vi "Init Master Slave Drive.vi"(0 "RobotDriveDevRef":T1={"DevStatus"={"status"=FALSE, "code"=0, "source"=""}, "Motors[]"=[], "Square Inputs"=FALSE, "Max Output"=1.0, "Isochronous"=FALSE}, 1 "Encoder Codes Per Rev":u16=64, 2 "Maximum Output Voltage":dbl=12.0, 3 "Encoder Initial Position":dbl format="%#_13g", 5 "Control Mode":T6=enum."Position", 7 "Left PID gains":T9={"proportional gain (Kp)"=1.0, "integral gain (Ki)"=0.01, "derivative gain (Kd)"=0.0}, 9 "Right PID gains":T9={"proportional gain (Kp)"=1.0, "integral gain (Ki)"=0.01, "derivative gain (Kd)"=0.0}, 11 "error in":errorcluster, 12 "Slave Mode":T6, 13 "Current Mode PID gains":T9={"proportional gain (Kp)"=1.0, "integral gain (Ki)"=0.01, "derivative gain (Kd)"=0.0}) -> (4 "RobotDriveDevRef Out":T1={"DevStatus"={"status"=FALSE, "code"=0, "source"=""}, "Motors[]"=[], "Square Inputs"=FALSE, "Max Output"=1.0, "Isochronous"=FALSE}, 15 "error out":errorcluster)   [LabVIEW 2013]
uses:
  <vilib>/Rock Robotics/WPI/RobotDrive/WPI_RobotDriveDevRef.ctl
  <vilib>/Rock Robotics/WPI/MotorControl/WPI_MotorControlDeviceRef.ctl
  <vilib>/Rock Robotics/SystemInterfaces/Typedef/FPGA_TypedefDigitalModule.ctl
  <vilib>/Rock Robotics/SystemInterfaces/DIO/FPGA_DIOPWMChannel.ctl
  <vilib>/Rock Robotics/WPI/PWM/WPI_PWMDeadband.ctl
  <vilib>/Rock Robotics/WPI/CAN/Jaguar/SubVIs/WPI_CANJaguar_ControlMode.ctl
  <vilib>/Rock Robotics/WPI/PWM/WPI_PWMTransform_ConPane.ctl
  <vilib>/Rock Robotics/WPI/CAN/Jaguar/SubVIs/WPI_CANJaguar_PositionReference.ctl
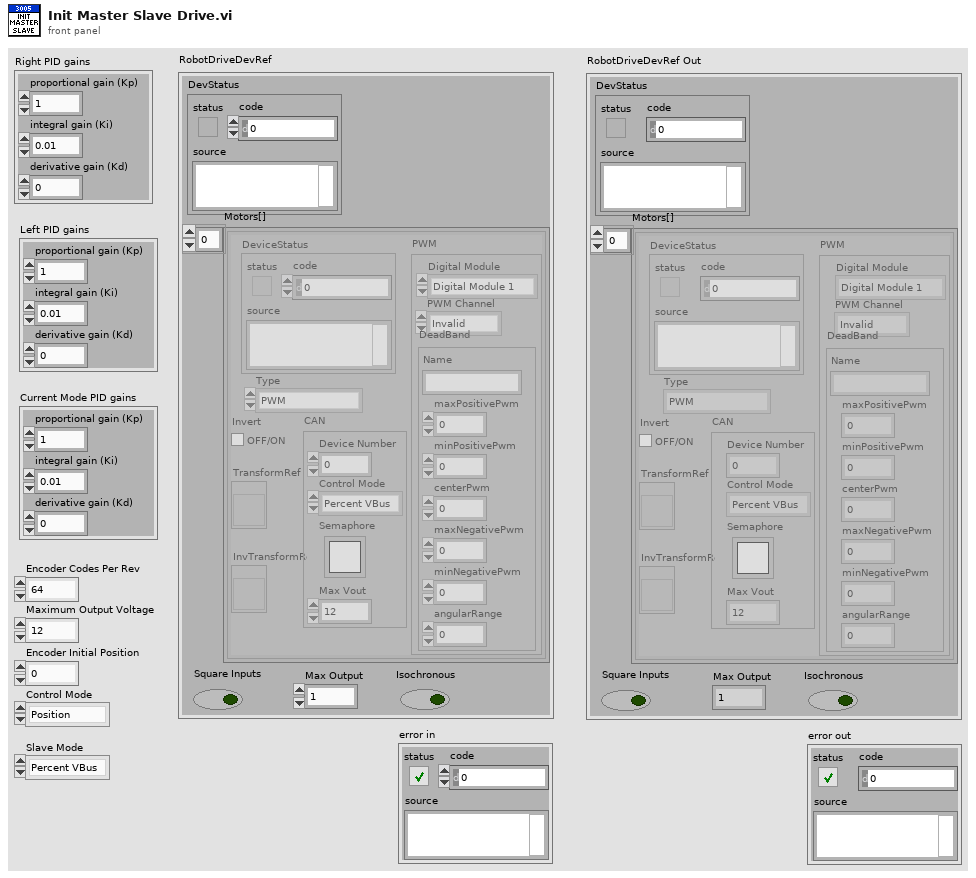
[diagram p1: front panel]
types:
  T1 = typedef "WPI_RobotDriveDevRef.ctl" = cluster{"DevStatus":errorcluster, "Motors[]":T2[], "Square Inputs":bool, "Max Output":dbl, "Isochronous":bool}
  T2 = typedef "WPI_MotorControlDeviceRef.ctl" = cluster{"DeviceStatus":errorcluster, "Type":enum16{"PWM", "CAN"}, "PWM":cluster{"Digital Module":T3, "PWM Channel":T4, "DeadBand":T5}, "CAN":cluster{"Device Number":u8, "Control Mode":T6, "Semaphore":T7, "Max Vout":dbl}, "Invert":bool, "TransformRef":T8, "InvTransformRef":T8}
  T3 = typedef "FPGA_TypedefDigitalModule.ctl" = enum16{"Digital Module 1", "Digital Module 2"}
  T4 = typedef "FPGA_DIOPWMChannel.ctl" = enum8{"PWM 1", "PWM 2", "PWM 3", "PWM 4", "PWM 5", "PWM 6", "PWM 7", "PWM 8", "PWM 9", "PWM 10", "Invalid"}
  T5 = typedef "WPI_PWMDeadband.ctl" = cluster{"Name":string, "maxPositivePwm":i32, "minPositivePwm":i32, "centerPwm":i32, "maxNegativePwm":i32, "minNegativePwm":i32, "angularRange":u16}
  T6 = typedef "WPI_CANJaguar_ControlMode.ctl" = enum8{"Percent VBus", "Current", "Speed", "Position", "Voltage"}
  T7 = typedef "Semaphore RefNum" = refnum<k1>
  T8 = typedef "WPI_PWMTransform_ConPane.ctl" = refnum<vi>
  T9 = cluster{"proportional gain (Kp)":dbl, "integral gain (Ki)":dbl, "derivative gain (Kd)":dbl}
  T10 = typedef "WPI_CANJaguar_PositionReference.ctl" = u8
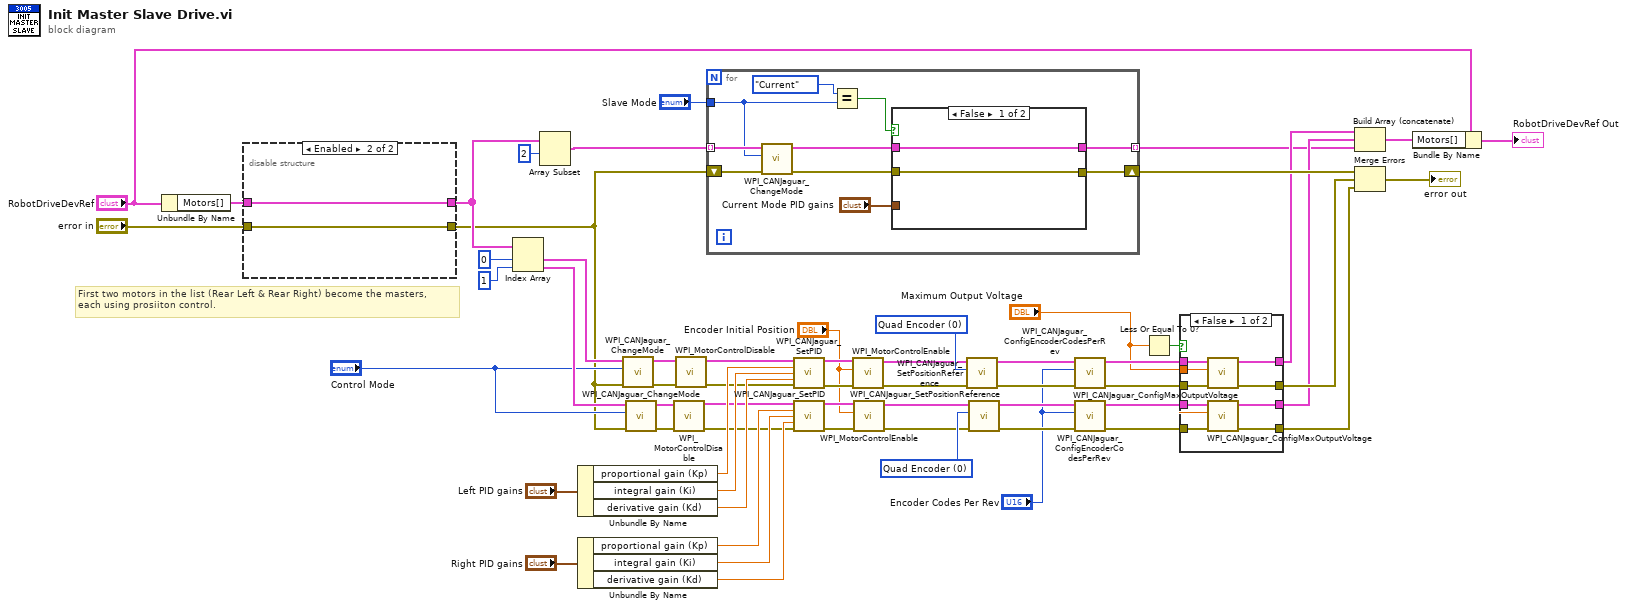
[diagram p0: block diagram]
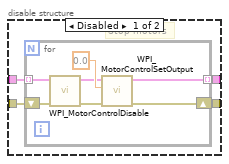
[diagram p2: hidden frame]
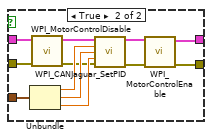
[diagram p3: hidden frame]
diagram:
  w48 = T10 0 items=["Quad Encoder"=0, "Potentiometer"=1, "None"=255] ("Position Reference")
  w49 = T10 0 items=["Quad Encoder"=0, "Potentiometer"=1, "None"=255] ("Position Reference")
  # "First two motors in the list (Rear Left & Rear Right) become the masters, \neach using prosiiton control."
  n1 = Unbundle By Name("RobotDriveDevRef") -> ("Motors[]"=w50:T2[])
  n2 = disable-structure shown="Enabled" {
    disable-tunnel: w50 -> [w64 w73]
    disable-tunnel: [w63 w73] -> w38
    disable-tunnel: "error in" -> [w62 w72]
    disable-tunnel: [w61 w72] -> w17
    frame Disabled {
      # "Stop motors"
      n3 = for {
        tunnel: w64 -> [w66] mode=indexing
        tunnel: [w68] -> w63 mode=indexing
        shift-right: [w69] -> w61
        shift-left: w62 -> [w70]
        n4 = call <vilib>:"WPI_MotorControlDisable.vi"("error in (no error)"=w70, "MotorControlDevRef"=w66) -> ("error out"=w67:errorcluster, "MotorControlDevRef"=w65:T2)  [unwired: 8 in]
        n5 = call <vilib>:"WPI_MotorControlSetOutput.vi"("error in (no error)"=w67, "Output"=0.0, "MotorControlDevRef"=w65) -> ("error out"=w69:errorcluster, "MotorControlDevRef"=w68:T2)  [unwired: 6 in, 1 out]
      }
    }
    frame Enabled {
    }
  }
  n6 = Index Array(array=w38, index #1=0 ("index"), index #2=1 ("index")) -> (element #1=w33:T2, element #2=w32:T2)
  n7 = Array Subset(array=w38, index=2) -> (w7:T2[])  [unwired: 1 in]
  n8 = Unbundle By Name("Left PID gains") -> ("proportional gain (Kp)"=w58:dbl, "integral gain (Ki)"=w57:dbl, "derivative gain (Kd)"=w56:dbl)
  n9 = Unbundle By Name("Right PID gains") -> ("proportional gain (Kp)"=w55:dbl, "integral gain (Ki)"=w54:dbl, "derivative gain (Kd)"=w53:dbl)
  n10 = call <vilib>:"WPI_CANJaguar_ChangeMode.vi"("error in (no error)"=w17, "Control Mode"="Control Mode", "CAN Jaguar Ref"=w33) -> ("error out"=w34:errorcluster, "CAN Jaguar Ref Out"=w15:T2)  [unwired: 7 in]
  n11 = call <vilib>:"WPI_CANJaguar_ChangeMode.vi"("error in (no error)"=w17, "Control Mode"="Control Mode", "CAN Jaguar Ref"=w32) -> ("error out"=w13:errorcluster, "CAN Jaguar Ref Out"=w12:T2)  [unwired: 7 in]
  n12 = call <vilib>:"WPI_MotorControlDisable.vi"("error in (no error)"=w13, "MotorControlDevRef"=w12) -> ("error out"=w10:errorcluster, "MotorControlDevRef"=w11:T2)  [unwired: 8 in]
  n13 = call <vilib>:"WPI_MotorControlDisable.vi"("error in (no error)"=w34, "MotorControlDevRef"=w15) -> ("error out"=w16:errorcluster, "MotorControlDevRef"=w14:T2)  [unwired: 8 in]
  n14 = for {
    tunnel: w7 -> [w83] mode=indexing
    shift-right: [w75] -> w23
    shift-left: w17 -> [w82]
    tunnel: "Slave Mode" -> [w80]
    tunnel: [w74] -> w4 mode=indexing
    n15 = call <vilib>:"WPI_CANJaguar_ChangeMode.vi"("error in (no error)"=w82, "Control Mode"=w80, "CAN Jaguar Ref"=w83) -> ("error out"=w77:errorcluster, "CAN Jaguar Ref Out"=w78:T2)  [unwired: 7 in]
    n16 = Equal?(x=WPI_CANJaguar_ControlMode."Current" ("y"), y=w80) -> (x = y?=w79:bool)
    n17 = case shown="False" w79 {
      tunnel: w78 -> [w85 w90]
      tunnel: w77 -> [w84 w97]
      tunnel: "Current Mode PID gains" -> [_ w95]
      tunnel: [w84 w88] -> w75
      tunnel: [w85 w86] -> w74
      frame False {
      }
      frame True {
        n18 = Unbundle(w95) -> ("proportional gain (Kp)"=w94:dbl, "integral gain (Ki)"=w93:dbl, "derivative gain (Kd)"=w92:dbl)
        n19 = call <vilib>:"WPI_MotorControlDisable.vi"("error in (no error)"=w97, "MotorControlDevRef"=w90) -> ("error out"=w91:errorcluster, "MotorControlDevRef"=w89:T2)  [unwired: 8 in]
        n20 = call <vilib>:"WPI_CANJaguar_SetPID.vi"("CAN Jaguar Ref"=w89, "P"=w94, "I"=w93, "D"=w92, "error in (no error)"=w91) -> ("CAN Jaguar Ref Out"=w87:T2, "error out"=w96:errorcluster)  [unwired: 9 in]
        n21 = call <vilib>:"WPI_MotorControlEnable.vi"("error in (no error)"=w96, "CAN Jaguar Ref"=w87) -> ("error out"=w88:errorcluster, "CAN Jaguar Ref Out"=w86:T2)  [unwired: 8 in]
      }
    }
  }
  n22 = call <vilib>:"WPI_CANJaguar_SetPID.vi"("CAN Jaguar Ref"=w14, "P"=w58, "I"=w57, "D"=w56, "error in (no error)"=w16) -> ("CAN Jaguar Ref Out"=w29:T2, "error out"=w36:errorcluster)  [unwired: 9 in]
  n23 = call <vilib>:"WPI_CANJaguar_SetPID.vi"("CAN Jaguar Ref"=w11, "P"=w55, "I"=w54, "D"=w53, "error in (no error)"=w10) -> ("CAN Jaguar Ref Out"=w26:T2, "error out"=w35:errorcluster)  [unwired: 9 in]
  n24 = call <vilib>:"WPI_MotorControlEnable.vi"("error in (no error)"=w36, "Encoder Initial Position"="Encoder Initial Position", "CAN Jaguar Ref"=w29) -> ("error out"=w30:errorcluster, "CAN Jaguar Ref Out"=w28:T2)  [unwired: 7 in]
  n25 = call <vilib>:"WPI_MotorControlEnable.vi"("error in (no error)"=w35, "Encoder Initial Position"="Encoder Initial Position", "CAN Jaguar Ref"=w26) -> ("error out"=w27:errorcluster, "CAN Jaguar Ref Out"=w25:T2)  [unwired: 7 in]
  n26 = call <vilib>:"WPI_CANJaguar_SetPositionReference.vi"("error in (no error)"=w30, "Position Reference"=w49, "CAN Jaguar Ref"=w28) -> ("error out"=w47:errorcluster, "CAN Jaguar Ref Out"=w44:T2)  [unwired: 7 in]
  n27 = call <vilib>:"WPI_CANJaguar_SetPositionReference.vi"("error in (no error)"=w27, "Position Reference"=w48, "CAN Jaguar Ref"=w25) -> ("error out"=w46:errorcluster, "CAN Jaguar Ref Out"=w45:T2)  [unwired: 7 in]
  n28 = call <vilib>:"WPI_CANJaguar_ConfigEncoderCodesPerRev.vi"("error in (no error)"=w47, "Encoder Codes Per Rev"="Encoder Codes Per Rev", "CAN Jaguar Ref"=w44) -> ("error out"=w42:errorcluster, "CAN Jaguar Ref Out"=w41:T2)  [unwired: 7 in]
  n29 = call <vilib>:"WPI_CANJaguar_ConfigEncoderCodesPerRev.vi"("error in (no error)"=w46, "Encoder Codes Per Rev"="Encoder Codes Per Rev", "CAN Jaguar Ref"=w45) -> ("error out"=w40:errorcluster, "CAN Jaguar Ref Out"=w39:T2)  [unwired: 7 in]
  n30 = Less Or Equal To 0?(x="Maximum Output Voltage") -> (x <= 0?=w19:bool)
  n31 = case shown="False" w19 {
    tunnel: w42 -> [w106 w110]
    tunnel: w41 -> [w105 w108]
    tunnel: w40 -> [w104 w109]
    tunnel: w39 -> [w103 w107]
    tunnel: "Maximum Output Voltage" -> [w102 _]
    tunnel: [w101 w110] -> w22
    tunnel: [w100 w109] -> w21
    tunnel: [w99 w108] -> w6
    tunnel: [w98 w107] -> w5
    frame False {
      n32 = call <vilib>:"WPI_CANJaguar_ConfigMaxOutputVoltage.vi"("error in (no error)"=w106, "Maximum Output Voltage"=w102, "CAN Jaguar Ref"=w105) -> ("error out"=w101:errorcluster, "CAN Jaguar Ref Out"=w99:T2)  [unwired: 7 in]
      n33 = call <vilib>:"WPI_CANJaguar_ConfigMaxOutputVoltage.vi"("error in (no error)"=w104, "Maximum Output Voltage"=w102, "CAN Jaguar Ref"=w103) -> ("error out"=w100:errorcluster, "CAN Jaguar Ref Out"=w98:T2)  [unwired: 7 in]
    }
    frame True {
    }
  }
  n34 = Build Array (concatenate)(w6, w5, w4) -> (w3:T2[])
  n35 = Merge Errors(w23, w22, w21) -> (→"error out":errorcluster)
  n36 = Bundle By Name(cluster="RobotDriveDevRef", "Motors[]"=w3) -> (→"RobotDriveDevRef Out":T1)
